vi "PascoPI.vi"(10 "Feedback":dbl, 11 "Setpoint":dbl) -> (3 "Motor Output":dbl)   [LabVIEW 2011]
panel:
  out "P Term":dbl(slide) scale=-1.0..1.0
  in  "Integrator Range":dbl=0.5
  out "I Term":dbl(slide) scale=-1.0..1.0
  in  "integral reset":bool
  in  "PID Out Max":dbl=1.0
  in  "?":T1={"P Gain"=0.1, "I Gain"=0.001, "D Gain"=0.0}
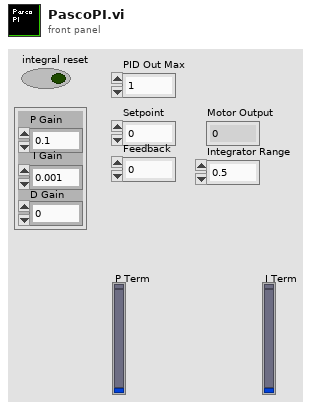
[diagram p1: front panel]
types:
  T1 = cluster{"P Gain":dbl, "I Gain":dbl, "D Gain":dbl}
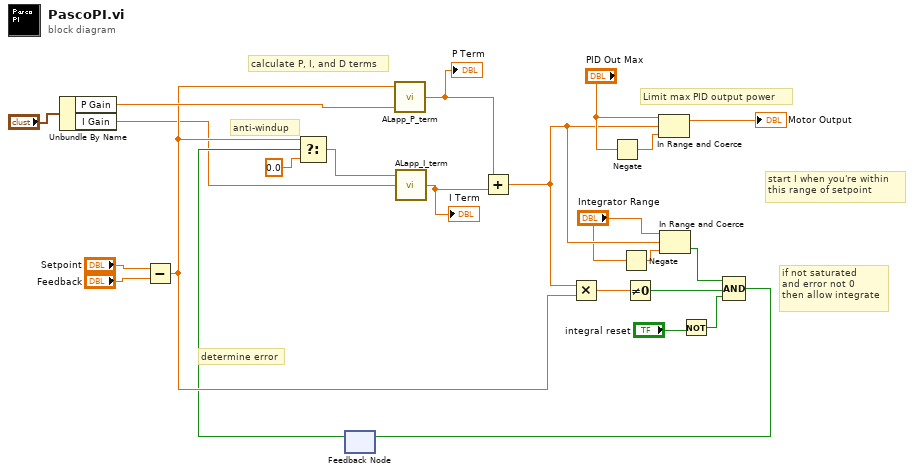
[diagram p0: block diagram]
diagram:
  # "start I when you're within \nthis range of setpoint"
  # "anti-windup"
  # "if not saturated\nand error not 0\nthen allow integrate"
  # "Limit max PID output power"
  # "calculate P, I, and D terms"
  # "determine error"
  n1 = Unbundle By Name("?") -> ("P Gain"=w16:dbl, "I Gain"=w8:dbl)
  n2 = Subtract(x="Setpoint", y="Feedback") -> (x-y=w14:dbl)
  n3 = feedback #1() -> (w12:bool)  [unwired: 1 out]
  n4 = Select(t=w14, s=w12, f=0.0) -> (s? t:f=w18:dbl)
  n5 = call "ALapp_P_term.vi"("P Term Gain"=w16, "Error"=w14) -> ("P Term"=w1:dbl)  [unwired: 1 out]
  "P Term" <- w1
  n6 = call "ALapp_I_term.vi"("I Term Gain"=w8, "error"=w18) -> ("I Term Output"=w19:dbl)  [unwired: 1 out]
  "I Term" <- w19
  n7 = Add(x=w1, y=w19) -> (x+y=w4:dbl)
  n8 = Multiply(x=w4, y=w14) -> (x*y=w11:dbl)
  n9 = Negate(x="PID Out Max") -> (-x=w21:dbl)
  n10 = Negate(x="Integrator Range") -> (-x=w2:dbl)
  n11 = Not Equal To 0?(x=w11) -> (x != 0?=w10:bool)
  n12 = In Range and Coerce(upper limit="PID Out Max", x=w4, lower limit=w21) -> (coerced(x)=→"Motor Output":dbl)  [unwired: 1 out]
  n13 = In Range and Coerce(upper limit="Integrator Range", x=w4, lower limit=w2) -> (In Range?=w5:bool)  [unwired: 1 out]
  n14 = Not(x="integral reset") -> (.not. x?=w6:bool)
  n15 = Compound Arithmetic op=AND(w5, w10, w6) -> (w13:bool)
  n16 = feedback-in #1(w13) -> ()
